vi "Read Background Mode.vi"(9 "Pane in":refnum<class "Pane.lvclass">) -> (3 "Pane out":refnum<class "Pane.lvclass">, 4 "Background Mode":enum16{"Stretch", "Center", "Tile"}(ring))   [LabVIEW 2014, in "Pane.lvclass"]
uses:
  Pane.lvclass
  Pane.lvclass/Pane.ctl
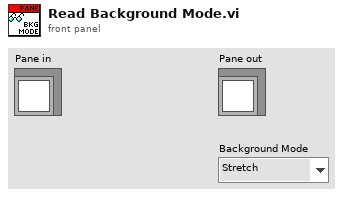
[diagram p1: front panel]
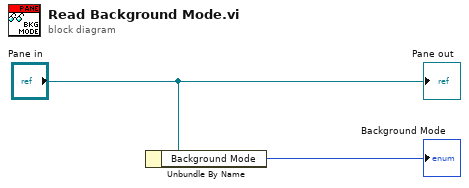
[diagram p0: block diagram]
diagram:
  n1 = Unbundle By Name("Pane in") -> ("Background Mode"=→"Background Mode":enum16{"Stretch", "Center", "Tile"})
  "Pane out" <- "Pane in"
